vi "MecaDriveKinematicsConstraint_getMaxVelocity.vi"(8 "Velocity":dbl, 9 "Curvature":dbl, 10 "statePose":T5={"TRANSLATION"={"X"=0.0, "Y"=0.0}, "ROTATION"={"VALUE"=0.0, "COS"=1.0, "SIN"=0.0}} {"ROTATION"."SIN" format="%13.4f"; "ROTATION"."COS" format="%13.4f"; "ROTATION"."VALUE" format="%13.4f"; "TRANSLATION"."Y" format="%14.3f"; "TRANSLATION"."X" format="%14.3f"}, 11 "MECANUM_DRIVE_KINE_CONSTRAINT":T1={"Max Speed (M/S)"=0.0, "MECA_DRIVE_KINEMATICS"={"FrontLeft"={"X"=0.0, "Y"=0.0}, "FrontRight"={"X"=0.0, "Y"=0.0}, "RearLeft"={"X"=0.0, "Y"=0.0}, "RearRight"={"X"=0.0, "Y"=0.0}, "InverseKinematics"=[[0.0, 1.0, -1.0, 0.0], [0.0, 1.0, 1.0, 0.0], [0.0, 1.0, 1.0, 0.0], [0.0, 1.0, -1.0, 0.0]], "ForwardKinematics"=[[0.0, 1.0, -1.0, 0.0], [0.0, 1.0, 1.0, 0.0], [0.0, 1.0, 1.0, 0.0], [0.0, 1.0, -1.0, 0.0]], "PrevCoR"={"X"=0.0, "Y"=0.0}}} {"MECA_DRIVE_KINEMATICS"."PrevCoR"."Y" format="%14.3f"; "MECA_DRIVE_KINEMATICS"."PrevCoR"."X" format="%14.3f"; "MECA_DRIVE_KINEMATICS"."RearRight"."Y" format="%14.3f"; "MECA_DRIVE_KINEMATICS"."RearRight"."X" format="%14.3f"; "MECA_DRIVE_KINEMATICS"."RearLeft"."Y" format="%14.3f"; "MECA_DRIVE_KINEMATICS"."RearLeft"."X" format="%14.3f"; "MECA_DRIVE_KINEMATICS"."FrontRight"."Y" format="%14.3f"; "MECA_DRIVE_KINEMATICS"."FrontRight"."X" format="%14.3f"; "MECA_DRIVE_KINEMATICS"."FrontLeft"."Y" format="%14.3f"; "MECA_DRIVE_KINEMATICS"."FrontLeft"."X" format="%14.3f"; "Max Speed (M/S)" format="%20.4f"}) -> (3 "absMaxVelocity":dbl)   [LabVIEW 2019, in "Trajectory_Library.lvlib"]
doc: "Return the maximum allowed velocity given the provided conditions.\n\n\nParameters:\n - MecanumDriveKinematicsConstraint - Constraint data structure\n - statePose - current traj state Pose\n - curvature - current traj curvature\n - maxVelocity - current traj max velocity\n\nReturns\n - maxVelocity - Maximum allowed velocity."
uses:
  Trajectory_Library.lvlib
  POSE2D.ctl
  TRANSLATION2D.ctl
  ROTATION2D.ctl
  TRAJ_CONSTRAINT_MECA_DRIVE_KINEMATICS.ctl
  MECA_DRIVE_KINEMATICS.ctl
  <vilib>/Analysis/Matrix/Datatypes/RealMatrix.ctl
  <vilib>/Analysis/Matrix/NI_Matrix.lvlib
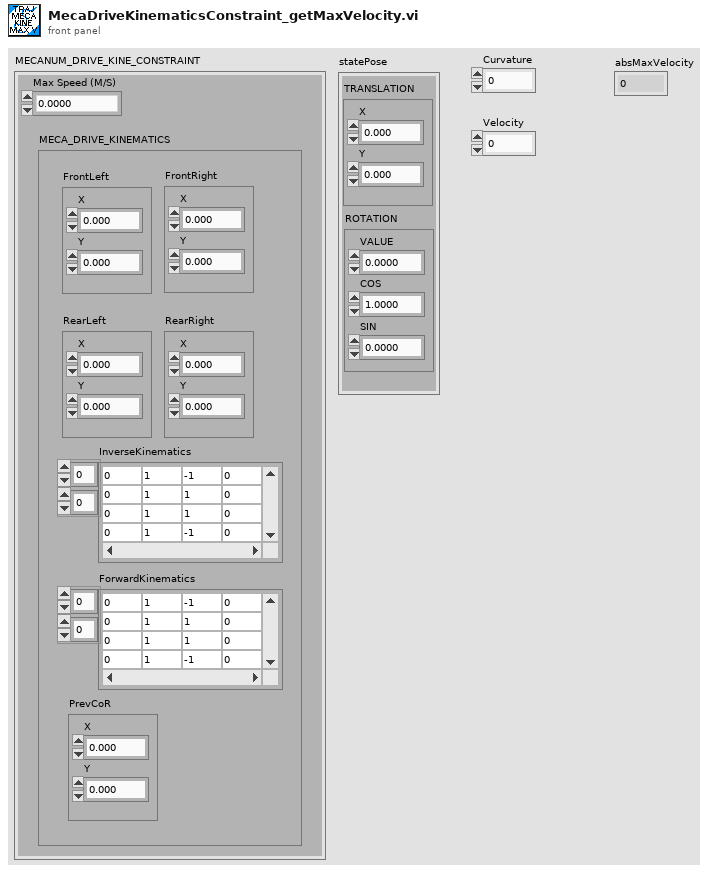
[diagram p1: front panel]
types:
  T1 = typedef "Trajectory_Library.lvlib/TRAJ_CONSTRAINT_MECA_DRIVE_KINEMATICS.ctl" = cluster{"Max Speed (M/S)":dbl, "MECA_DRIVE_KINEMATICS":T2}
  T2 = typedef "Trajectory_Library.lvlib/MECA_DRIVE_KINEMATICS.ctl" = cluster{"FrontLeft":T3, "FrontRight":T3, "RearLeft":T3, "RearRight":T3, "InverseKinematics":T4, "ForwardKinematics":T4, "PrevCoR":T3}
  T3 = typedef "Trajectory_Library.lvlib/TRANSLATION2D.ctl" = cluster{"X":dbl, "Y":dbl}
  T4 = typedef "NI_Matrix.lvlib/RealMatrix.ctl" = dbl[][]
  T5 = typedef "Trajectory_Library.lvlib/POSE2D.ctl" = cluster{"TRANSLATION":T3, "ROTATION":T6}
  T6 = typedef "Trajectory_Library.lvlib/ROTATION2D.ctl" = cluster{"VALUE":dbl, "COS":dbl, "SIN":dbl}
  T7 = typedef "Trajectory_Library.lvlib/CHASSIS_SPEEDS.ctl" = cluster{"vX":dbl, "vY":dbl, "vOmega":dbl}
  T8 = typedef "Trajectory_Library.lvlib/MECA_WHEEL_SPEEDS.ctl" = cluster{"FrontLeftSpeed":dbl, "FrontRightSpeed":dbl, "RearLeftSpeed":dbl, "RearRightSpeed":dbl}
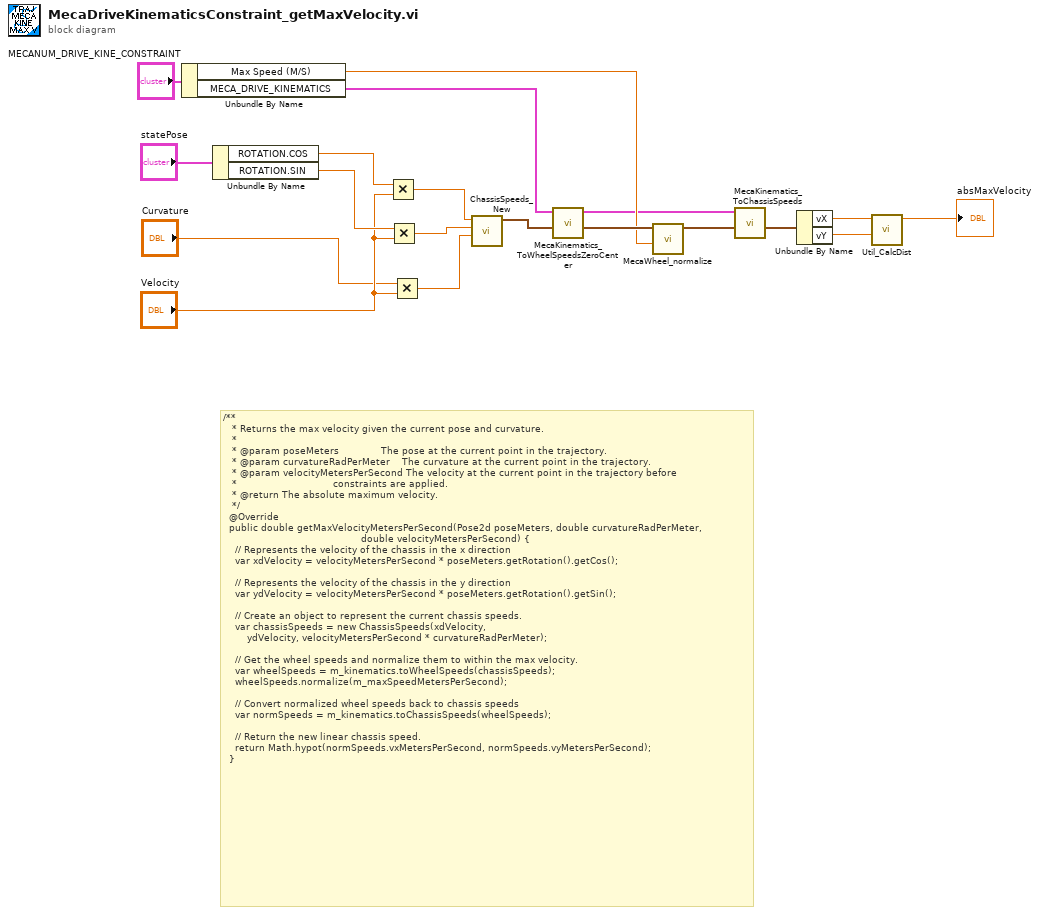
[diagram p0: block diagram]
diagram:
  # "/**\n   * Returns the max velocity given the current pose and curvature.\n   *\n   * @param poseMeters              The pose at the current point in the trajectory.\n   * @param curvatureRadPerMeter    The curvature at the current point in the trajectory.\n   * @param velocityMetersPerSecond The velocity at the current point in the trajectory before\n   *                                constraints are applied.\n   * @return The absolute maximum velocity.\n   */\n  @Override\n  public double getMaxVelocityMetersPerSecond(Pose2d poseMeters, double curvatureRadPerMeter,\n                                              double velocityMetersPerSecond) {\n    // Represents the velocity of the chassis in the x direction\n    var xdVelocity = velocityMetersPerSecond * poseMeters.getRotation().getCos();\n\n    // Represents the velocity of the chassis in the y direction\n    var ydVelocity = velocityMetersPerSecond * poseMeters.getRotation().getSin();\n\n    // Create an object to represent the current chassis speeds.\n    var chassisSpeeds = new ChassisSpeeds(xdVelocity,\n        ydVelocity, velocityMetersPerSecond * curvatureRadPerMeter);\n\n    // Get the wheel speeds and normalize them to within the max velocity.\n    var wheelSpeeds = m_kinematics.toWheelSpeeds(chassisSpeeds);\n    wheelSpeeds.normalize(m_maxSpeedMetersPerSecond);\n\n    // Convert normalized wheel speeds back to chassis speeds\n    var normSpeeds = m_kinematics.toChassisSpeeds(wheelSpeeds);\n\n    // Return the new linear chassis speed.\n    return Math.hypot(normSpeeds.vxMetersPerSecond, normSpeeds.vyMetersPerSecond);\n  }"
  n1 = Unbundle By Name("MECANUM_DRIVE_KINE_CONSTRAINT") -> ("Max Speed (M/S)"=w9:dbl, "MECA_DRIVE_KINEMATICS"=w2:T2)
  n2 = Unbundle By Name("statePose") -> ("ROTATION.COS"=w18:dbl, "ROTATION.SIN"=w17:dbl)
  n3 = Multiply(x=w18, y="Velocity") -> (x*y=w14:dbl)
  n4 = Multiply(x=w17, y="Velocity") -> (x*y=w13:dbl)
  n5 = Multiply(x="Curvature", y="Velocity") -> (x*y=w12:dbl)
  n6 = call "ChassisSpeeds_New.vi"("vAngular"=w12, "vY"=w13, "vX"=w14) -> ("CHASSIS"=w1:T7)  [unwired: 8 in]
  n7 = call "MecaKinematics_ToWheelSpeedsZeroCenter.vi"("ChassisSpeeds"=w1, "in MECA_DRIVE_KINEMATICS"=w2) -> ("MECA_WHEEL_SPEEDS"=w10:T8, "out MECA_DRIVE_KINEMATICS"=w7:T2)  [unwired: 8 in]
  n8 = call "MecaWheel_normalize.vi"("MaxAttainableSpeed"=w9, "in MECA_WHEEL_SPEEDS"=w10) -> ("out MECA_WHEEL_SPEEDS"=w8:T8)  [unwired: 9 in]
  n9 = call "MecaKinematics_ToChassisSpeeds.vi"("MECA_WHEEL_SPEEDS"=w8, "in MECA_DRIVE_KINEMATICS"=w7) -> ("ChassisSpeeds"=w6:T7)  [unwired: 9 in]
  n10 = Unbundle By Name(w6) -> ("vX"=w5:dbl, "vY"=w4:dbl)
  n11 = call "Util_CalcDist.vi"("Y"=w4, "X"=w5) -> ("DIST"=→"absMaxVelocity":dbl)  [unwired: 9 in]
